vi "VISA query.vi"(7 "timeout(ms)":i32=500, 8 "error in":errorcluster, 9 "delay(ms)":i32=50, 10 "write buffer":string, 11 "VISA resource name":refnum<visa-resource-name>) -> (0 "error out":errorcluster, 2 "read buffer":string, 3 "VISA resource name out":refnum<visa-resource-name>)   [LabVIEW 2014]
panel:
  out "return count":u32
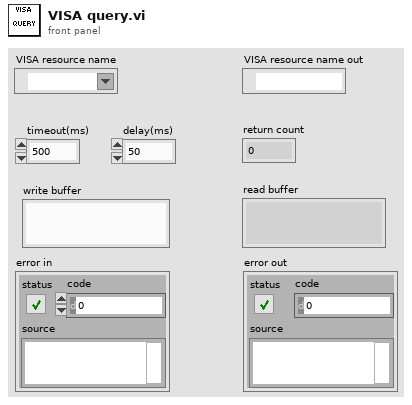
[diagram p1: front panel]
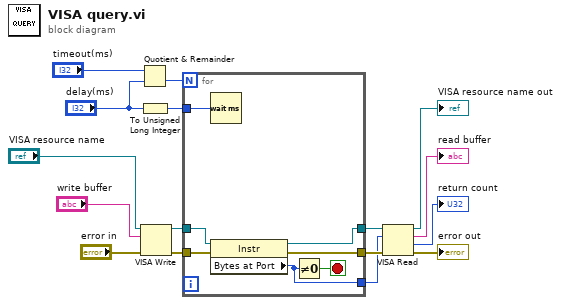
[diagram p0: block diagram]
diagram:
  n1 = Quotient & Remainder(x="timeout(ms)", y="delay(ms)") -> (floor(x/y)=w2:i32)  [unwired: 1 out]
  n2 = To Unsigned Long Integer(number="delay(ms)") -> (unsigned 32bit integer=w1:u32)
  n3 = VISA Write(VISA resource name="VISA resource name", write buffer="write buffer", error in (no error)="error in") -> (VISA resource name out=w14:refnum<visa-resource-name>, error out=w13:errorcluster)  [unwired: 1 out]
  n4 = for {
    N: w2 -> [_]
    tunnel: [w20] -> w12
    tunnel: [w23] -> w16
    tunnel: [w22] -> w15
    tunnel: w14 -> [w19]
    tunnel: w13 -> [w18]
    tunnel: w1 -> [w17]
    stop <- w21 stop-if-true
    n5 = Wait (ms)(milliseconds to wait=w17) -> ()  [unwired: 1 out]
    n6 = property class="Instr"(reference=w19, error in=w18) -> (reference out=w23:refnum<visa-resource-name>, error out=w22:errorcluster, "Bytes at Port"=w20:u32)
    n7 = Not Equal To 0?(x=w20) -> (x != 0?=w21:bool)
  }
  n8 = VISA Read(VISA resource name=w16, byte count=w12, error in (no error)=w15) -> (VISA resource name out=→"VISA resource name out":refnum<visa-resource-name>, read buffer=→"read buffer":string, return count=→"return count":u32, error out=→"error out":errorcluster)
